vi "createElement.vi"(6 "collectionInfo":T1, 8 "error in (no error)":errorcluster, 9 "elementBasicType":string, 10 "elementName":string, 11 "IElementFactory in":refnum<class "IElementFactory.lvclass">) -> (0 "error out":errorcluster, 2 "element":refnum<class "Element.lvclass">, 3 "IElementFactory out":refnum<class "IElementFactory.lvclass">)   [LabVIEW 2016, in "IElementFactory.lvclass"]
uses:
  IElementFactory.lvclass
  Element/Element.lvclass
  Typedefs/CollectionInfo.ctl
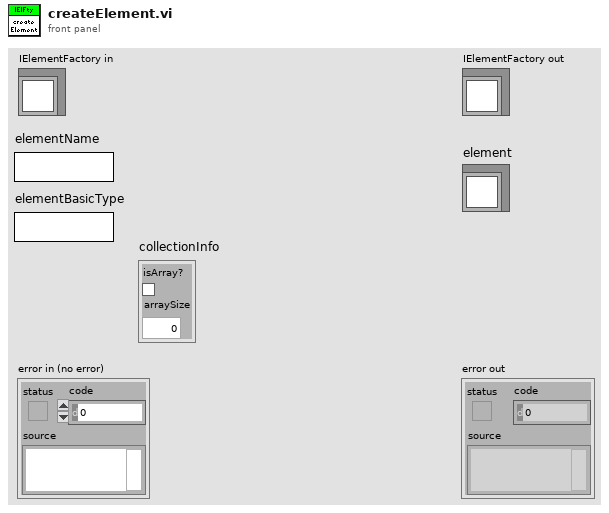
[diagram p1: front panel]
types:
  T1 = typedef "CollectionInfo.ctl" = cluster{"isArray?":bool, "arraySize":u16}
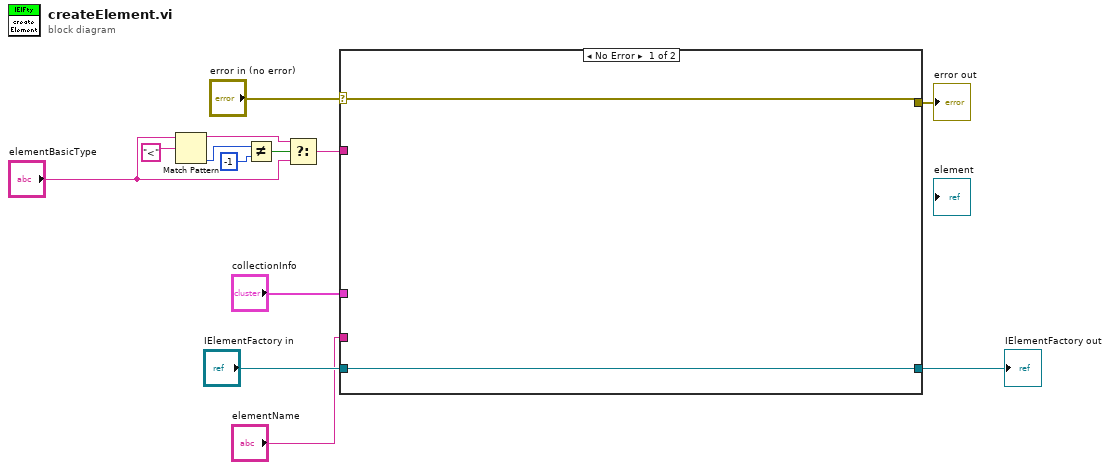
[diagram p0: block diagram]
diagram:
  n1 = Match Pattern(string="elementBasicType", regular expression="<") -> (before substring=w3:string, offset past match=w6:i32)  [unwired: 1 in, 2 out]
  n2 = Not Equal?(x=w6, y=-1) -> (x != y?=w4:bool)
  n3 = Select(t=w3, s=w4, f="elementBasicType") -> (s? t:f=w1:string)
  n4 = case shown="No Error" "error in (no error)" {
    selector: "error in (no error)" -> [w14 w17]
    tunnel: [w14 w17] -> w12
    tunnel: [w15 w16] -> w10
    tunnel: "IElementFactory in" -> [w15 w16]
    tunnel: w1 -> [_ _]
    tunnel: "collectionInfo" -> [_ _]
    tunnel: "elementName" -> [_ _]
    frame No Error {
    }
    frame Error {
    }
  }
  "error out" <- w12
  "IElementFactory out" <- w10
